vi "box catch_old_1.vi"(8 "error in (no error)":errorcluster, 9 "now position":cluster{"x":dbl, "y":dbl, "degree":dbl}) -> (0 "error out":errorcluster, 1 "position out":cluster{"x":dbl, "y":dbl, "degree":dbl})   [LabVIEW 2019]
uses:
  ctl/continued move array-V2.ctl
  servo state.ctl
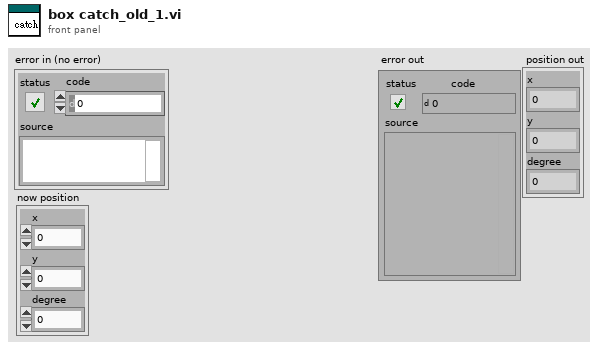
[diagram p1: front panel]
types:
  T1 = typedef "servo state.ctl" = enum16{"catch", "cam-1", "put", "side", "center", "side-2"}
  T2 = typedef "continued move array-V2.ctl" = cluster{"X":dbl, "Y":dbl, "Speed":dbl, "rotate\ndegree":dbl, "deg":dbl}
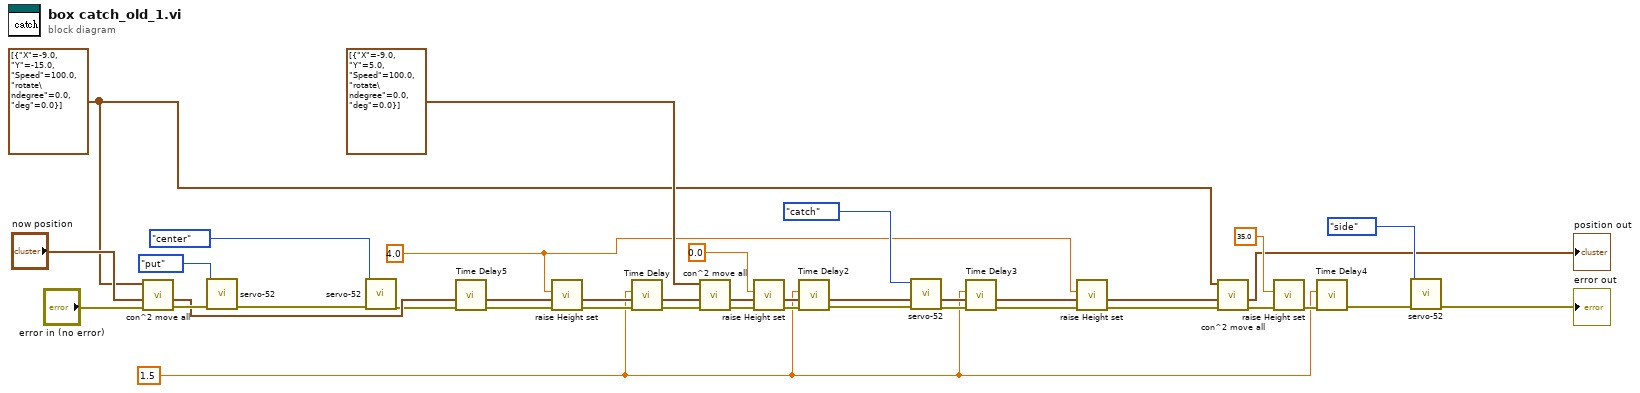
[diagram p0: block diagram]
diagram:
  w7 = 1.5
  w4 = 4.0 ("Height_cm")
  w15 = T2[] [{"X"=-9.0, "Y"=-15.0, "Speed"=100.0, "rotate\ndegree"=0.0, "deg"=0.0}] ("contrast move array")
  n1 = call "con^2 move all.vi"("error in (no error)"="error in (no error)", "now position"="now position", "contrast move array"=w15) -> ("error out"=w30:errorcluster, "position out"=w27:cluster{"x":dbl, "y":dbl, "degree":dbl})  [unwired: 7 in]
  n2 = call "servo-52.vi"("error in (no error)"=w30, "Enum"=servo_state."put") -> ("error out"=w1:errorcluster)  [unwired: 9 in]
  n3 = call "servo-52.vi"("error in (no error)"=w1, "Enum"=servo_state."center") -> ("error out"=w2:errorcluster)  [unwired: 9 in]
  n4 = call "Time Delay5"("error in (no error)"=w2) -> ("error out"=w3:errorcluster)  [unwired: 10 in]
  n5 = call "raise Height set.vi"("error in (no error)"=w3, "Height_cm"=w4) -> ("error out"=w26:errorcluster)  [unwired: 9 in]
  n6 = call "Time Delay"("error in (no error)"=w26, "Delay Time (s)"=w7) -> ("error out"=w25:errorcluster)  [unwired: 9 in]
  n7 = call "con^2 move all.vi"("error in (no error)"=w25, "now position"=w27, "contrast move array"=T2[] [{"X"=-9.0, "Y"=5.0, "Speed"=100.0, "rotate\ndegree"=0.0, "deg"=0.0}]) -> ("error out"=w22:errorcluster, "position out"=w16:cluster{"x":dbl, "y":dbl, "degree":dbl})  [unwired: 7 in]
  n8 = call "raise Height set.vi"("error in (no error)"=w22, "Height_cm"=0.0) -> ("error out"=w20:errorcluster)  [unwired: 9 in]
  n9 = call "Time Delay2"("error in (no error)"=w20, "Delay Time (s)"=w7) -> ("error out"=w19:errorcluster)  [unwired: 9 in]
  n10 = call "servo-52.vi"("error in (no error)"=w19, "Enum"=servo_state."catch") -> ("error out"=w17:errorcluster)  [unwired: 9 in]
  n11 = call "Time Delay3"("error in (no error)"=w17, "Delay Time (s)"=w7) -> ("error out"=w5:errorcluster)  [unwired: 9 in]
  n12 = call "raise Height set.vi"("error in (no error)"=w5, "Height_cm"=w4) -> ("error out"=w6:errorcluster)  [unwired: 9 in]
  n13 = call "con^2 move all.vi"("error in (no error)"=w6, "now position"=w16, "contrast move array"=w15) -> ("error out"=w14:errorcluster, "position out"=→"position out":cluster{"x":dbl, "y":dbl, "degree":dbl})  [unwired: 7 in]
  n14 = call "raise Height set.vi"("error in (no error)"=w14, "Height_cm"=35.0) -> ("error out"=w12:errorcluster)  [unwired: 9 in]
  n15 = call "Time Delay4"("error in (no error)"=w12, "Delay Time (s)"=w7) -> ("error out"=w11:errorcluster)  [unwired: 9 in]
  n16 = call "servo-52.vi"("error in (no error)"=w11, "Enum"=servo_state."side") -> ("error out"=→"error out":errorcluster)  [unwired: 9 in]
